vi "Set Data.vi"(8 "error in (no error)":errorcluster, 9 "Data":variant, 10 "Name":string, 11 "Dictionary in":refnum<class "Dictionary.lvclass">) -> (0 "error out":errorcluster, 3 "Dictionary out":refnum<class "Dictionary.lvclass">)   [LabVIEW 2014, in "bmlv.lvlib" / "Dictionary.lvclass"]
uses:
  Dictionary.lvclass
  Dictionary.lvclass/Dictionary.ctl
  Read Dict.vi
  Write Dict.vi
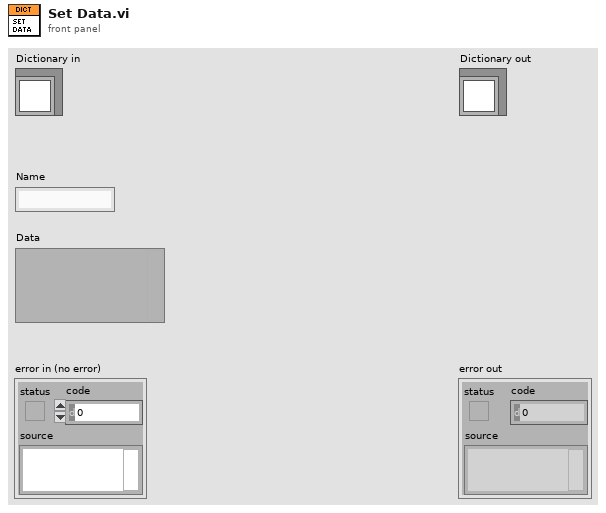
[diagram p1: front panel]
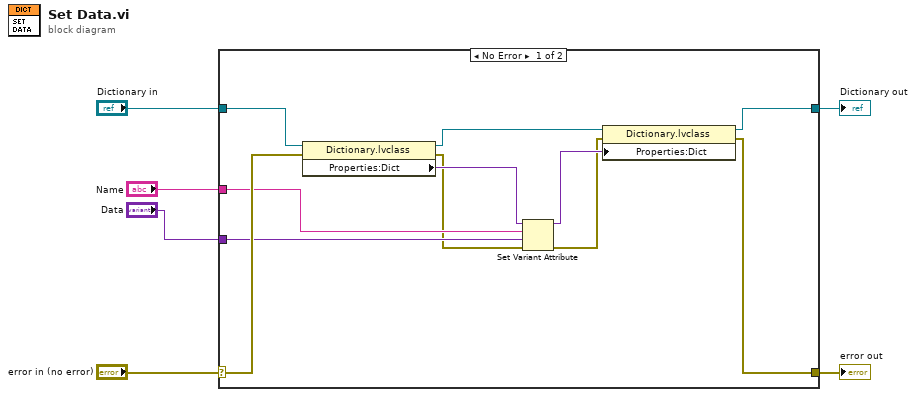
[diagram p0: block diagram]
diagram:
  n1 = case shown="No Error" "error in (no error)" {
    selector: "error in (no error)" -> [w16 w19]
    tunnel: [w7 w19] -> w5
    tunnel: [w8 w18] -> w3
    tunnel: "Dictionary in" -> [w17 w18]
    tunnel: "Name" -> [w14 _]
    tunnel: "Data" -> [w13 _]
    frame No Error {
      n2 = property class="Dictionary.lvclass"(reference=w17, error in=w16) -> (reference out=w11:refnum<class "Dictionary.lvclass">, error out=w12:errorcluster, "Properties:Dict"=w15:variant)
      n3 = Set Variant Attribute(Variant=w15, name=w14, value=w13, error in=w12) -> (Variant out=w10:variant, error out=w9:errorcluster)  [unwired: 1 out]
      n4 = property class="Dictionary.lvclass"(reference=w11, error in=w9, "Properties:Dict"=w10) -> (reference out=w8:refnum<class "Dictionary.lvclass">, error out=w7:errorcluster)
    }
    frame Error {
    }
  }
  "error out" <- w5
  "Dictionary out" <- w3
